vi "Read Pin Map.vi"(8 "error in (no error)":errorcluster, 11 "Arduino in":refnum<class "Arduino.lvclass">) -> (0 "error out":errorcluster, 2 "Pin Map":T1={"Region Valves"=[49, 52, 0, 0], "Extra Valves"=[[[0.0, 48.0, 0.0, 0.0, 0.0]]], "Tool Primary Valve"=51, "Tool Secondary Valve"=50, "Region Sensors"=[37, 41, 37], "Extra Sensors"=[[[36.0, 37.0, 0.0, 0.0]]], "Tool Primary Sensor"=39.0, "Tool Secondary Sensor"=38.0, "Compression Sensor"=31.0, "5V"=50, "Dispenser Sensor"=0.0, "Light Curtain"=50}, 3 "Arduino out":refnum<class "Arduino.lvclass">)   [LabVIEW 2021, in "Arduino.lvclass"]
uses:
  Arduino.lvclass
  Pin Map.ctl
  I-O.lvclass
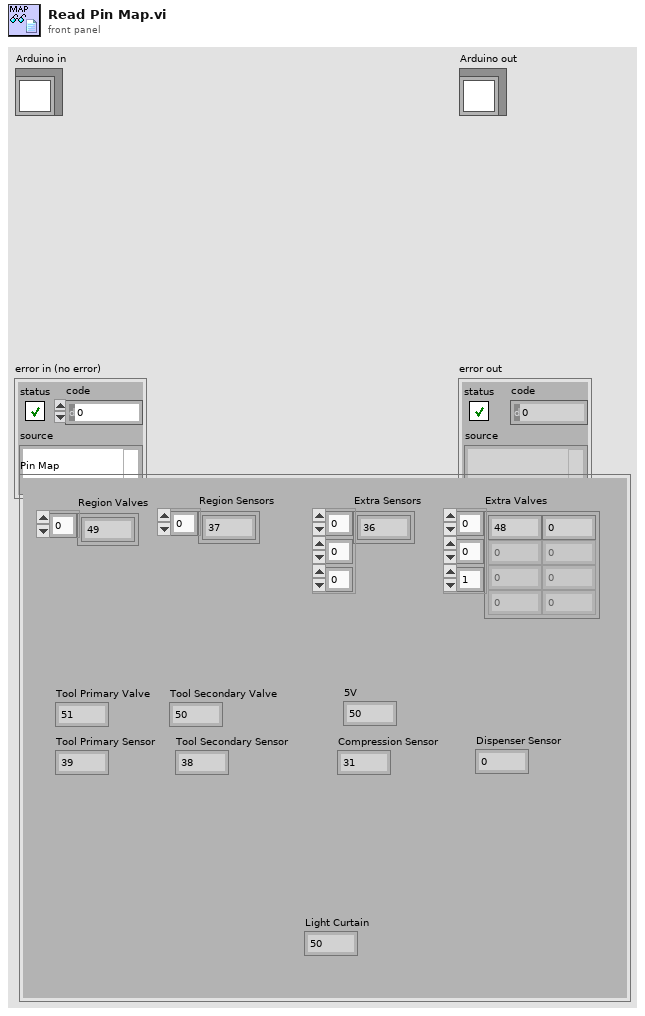
[diagram p1: front panel]
types:
  T1 = typedef "I-O.lvclass/Pin Map.ctl" = cluster{"Region Valves":i32[], "Extra Valves":dbl[][][], "Tool Primary Valve":i32, "Tool Secondary Valve":i32, "Region Sensors":i32[], "Extra Sensors":dbl[][][], "Tool Primary Sensor":dbl, "Tool Secondary Sensor":dbl, "Compression Sensor":dbl, "5V":i32, "Dispenser Sensor":dbl, "Light Curtain":i32}
  T2 = typedef "I-O.lvclass/Pin Map.ctl" = cluster{"Region Valves":i32[], "Extra Valves":dbl[][][], "Tool Primary Valve":i32, "Tool Secondary Valve":i32, "Region Sensors":i32[], "Extra Sensors":dbl[][][], "Tool Primary Sensor":dbl, "Tool Secondary Sensor":dbl, "Compression Sensor":dbl, "5V":i32}
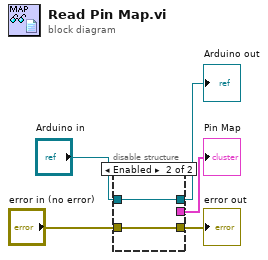
[diagram p0: block diagram]
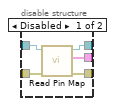
[diagram p2: hidden frame]
diagram:
  n1 = disable-structure shown="Enabled" {
    disable-tunnel: [w10 w12] -> w5
    disable-tunnel: [w9 w11] -> w4
    disable-tunnel: "error in (no error)" -> [w8 w12]
    disable-tunnel: "Arduino in" -> [w7 w11]
    disable-tunnel: [w6 _] -> w1
    frame Disabled {
      n2 = call-parent "Read Pin Map.vi"("error in (no error)"=w8, "I-O in"=w7) -> ("error out"=w10:errorcluster, "Pin Map 2"=w6:T2, "I-O out"=w9:refnum<class "Arduino.lvclass">)  [unwired: 7 in]
    }
    frame Enabled {
    }
  }
  "error out" <- w5
  "Arduino out" <- w4
  "Pin Map" <- w1
